vi "SortIconsInNameOrder.vi"(9 "Icons File Order":picture[](array[picture]), 10 "File Order":string[](array[string]), 11 "Name Order":string[](array[string])) -> (1 "Order":i32[](array[numeric]), 2 "Icons names":string[](array[string]), 3 "Icons name order":picture[](array[picture]))   [LabVIEW 2022 SP3]
doc: "This VI sorts <b>Icons File Order</b> array (arranged by <b>File Order</b> names) according to <b>Name Order</b>. \n\n<b>Icons File Order</b> - Input Array of Icons in File order. \n<b>File Order</b> - Input order of the Icons names in Icons File Order. \n<b>Name Order</b> - Input of the required order of Icons. \n<b>Icons names</b> - An output array of sorted names according to Name Order. \n<b>Order</b> - Output of the search Indexes of each element in Name Order in File Order"
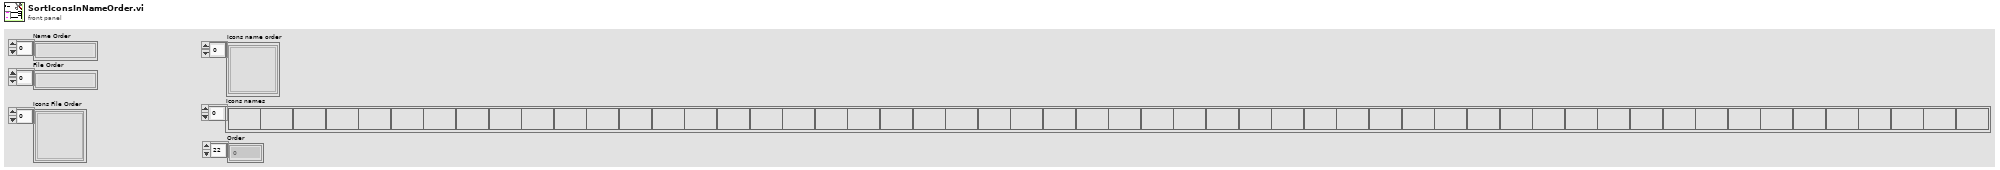
[diagram p1: front panel]
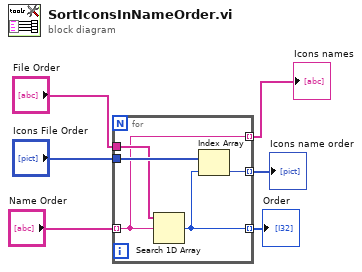
[diagram p0: block diagram]
diagram:
  n1 = for {
    tunnel: "Icons File Order" -> [w11]
    tunnel: [w10] -> w5 mode=indexing
    tunnel: "File Order" -> [w9]
    tunnel: "Name Order" -> [w7] mode=indexing
    tunnel: [w8] -> w2 mode=indexing
    tunnel: [w7] -> w1 mode=indexing
    n2 = Search 1D Array(1D array=w9, element=w7) -> (index of element=w8:i32)  [unwired: 1 in]
    n3 = Index Array(array=w11, index=w8) -> (element=w10:picture)
  }
  "Icons names" <- w1
  "Icons name order" <- w5
  "Order" <- w2
